vi "Asylum_SetPISLoop.vi"(5 "whichLoop":i32, 6 "outChannelString":string, 7 "eventString":string, 8 "error in (no error)":errorcluster, 9 "PIS Controls":T1, 10 "inChannelString":string, 11 "Application":refnum<k7>) -> (0 "error out":errorcluster, 3 "Application":refnum<k7>)   [LabVIEW 2016]
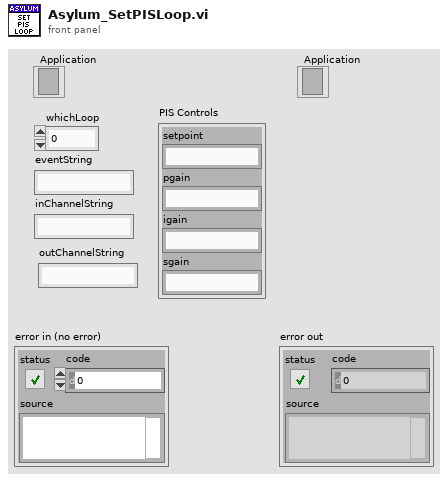
[diagram p1: front panel]
types:
  T1 = cluster{"setpoint":string, "pgain":string, "igain":string, "sgain":string}
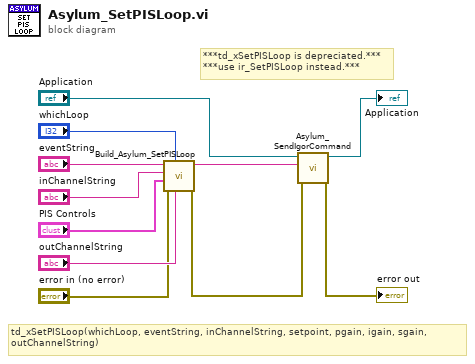
[diagram p0: block diagram]
diagram:
  # "***td_xSetPISLoop is depreciated.***\n***use ir_SetPISLoop instead.***"
  # "td_xSetPISLoop(whichLoop, eventString, inChannelString, setpoint, pgain, igain, sgain,\noutChannelString)"
  n1 = call "Build_Asylum_SetPISLoop.vi"("outChannelString"="outChannelString", "whichLoop"="whichLoop", "error in (no error)"="error in (no error)", "PIS Controls"="PIS Controls", "inChannelString"="inChannelString", "eventString"="eventString") -> ("error out"=w1:errorcluster, "Command"=w9:string)  [unwired: 4 in]
  n2 = call "Asylum_SendIgorCommand.vi"("error in (no error)"=w1, "command"=w9, "Application"="Application") -> ("error out"=→"error out":errorcluster, "Application"=→"Application":refnum<k7>)  [unwired: 5 in, 2 out]
